vi "apply data indices.vi"(8 "error in":errorcluster, 10 "index type defs":T1, 11 "Temperature Chamber Model runtime in":refnum<class "Temperature Chamber Model runtime.lvclass">) -> (0 "error out":errorcluster, 3 "Temperature Chamber Model runtime out":refnum<class "Temperature Chamber Model runtime.lvclass">)   [LabVIEW 2013, in "Temperature Chamber Model runtime.lvclass"]
uses:
  Temperature Chamber Model runtime.lvclass
  <vilib>/NI/Tag Bus Data Framework/fixed module parent/module/configuration/index type definitions.ctl
  configuration/input data indices.ctl
  configuration/output data indices.ctl
  configuration/parameter data indices.ctl
  configuration/result data indices.ctl
  Temperature Chamber Model runtime.lvclass/Temperature Chamber Model runtime.ctl
  configuration/Temperature Chamber Model configuration.lvclass
  <vilib>/NI/Tag Bus Data Framework/fixed module parent/module/configuration/fixed channel configuration.lvclass
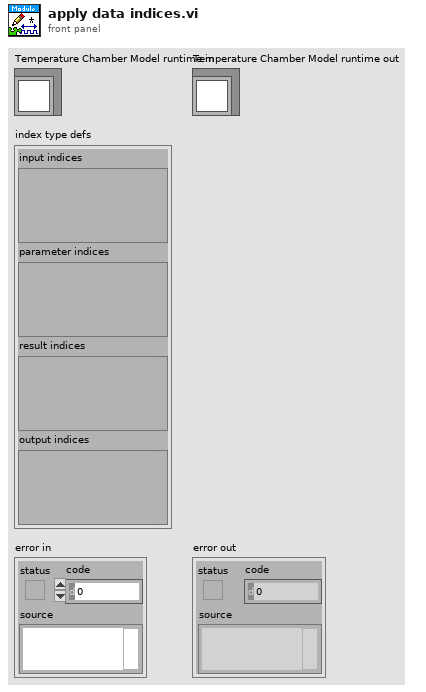
[diagram p1: front panel]
types:
  T1 = typedef "fixed channel configuration.lvclass/index type definitions.ctl" = cluster{"input indices":variant, "parameter indices":variant, "result indices":variant, "output indices":variant}
  T2 = typedef "Temperature Chamber Model configuration.lvclass/result data indices.ctl" = cluster{"Double.Thermocouple Reading":i32}
  T3 = typedef "Temperature Chamber Model configuration.lvclass/parameter data indices.ctl" = cluster{"Double.Ambient Temperature":i32, "Double.Fan PWM":i32, "Double.Lamp PWM":i32}
  T4 = typedef "Temperature Chamber Model configuration.lvclass/output data indices.ctl" = cluster{"fmwk_placeholder":i32}
  T5 = typedef "Temperature Chamber Model configuration.lvclass/input data indices.ctl" = cluster{"fmwk_placeholder":i32}
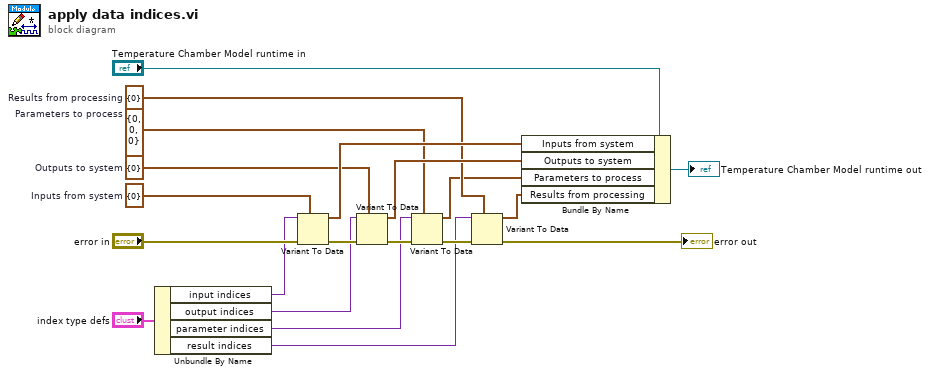
[diagram p0: block diagram]
diagram:
  w3 = T2 {"Double.Thermocouple Reading"=0}  # Results from processing
  w4 = T3 {"Double.Ambient Temperature"=0, "Double.Fan PWM"=0, "Double.Lamp PWM"=0}  # Parameters to process
  w8 = T4 {"fmwk_placeholder"=0}  # Outputs to system
  w11 = T5 {"fmwk_placeholder"=0}  # Inputs from system
  n1 = Unbundle By Name("index type defs") -> ("input indices"=w12:variant, "output indices"=w9:variant, "parameter indices"=w6:variant, "result indices"=w5:variant)
  n2 = Variant To Data(error in="error in", type=w11, Variant=w12) -> (data=w10:T5, error out=w13:errorcluster)
  n3 = Variant To Data(error in=w13, type=w8, Variant=w9) -> (data=w7:T4, error out=w16:errorcluster)
  n4 = Variant To Data(error in=w16, type=w4, Variant=w6) -> (data=w2:T3, error out=w14:errorcluster)
  n5 = Variant To Data(error in=w14, type=w3, Variant=w5) -> (data=w1:T2, error out=→"error out":errorcluster)
  n6 = Bundle By Name(cluster="Temperature Chamber Model runtime in", "Inputs from system"=w10, "Outputs to system"=w7, "Parameters to process"=w2, "Results from processing"=w1) -> (→"Temperature Chamber Model runtime out":refnum<class "Temperature Chamber Model runtime.lvclass">)
